vi "destroy.vi"(8 "error in (no error)":errorcluster, 11 "OvenController in":refnum<class "OvenController.lvclass">) -> (0 "error out":errorcluster)   [LabVIEW 2023, in "AbstractFactory.lvlib" / "OvenController.lvclass"]
uses:
  OvenController.lvclass
  OvenController.lvclass/OvenController.ctl
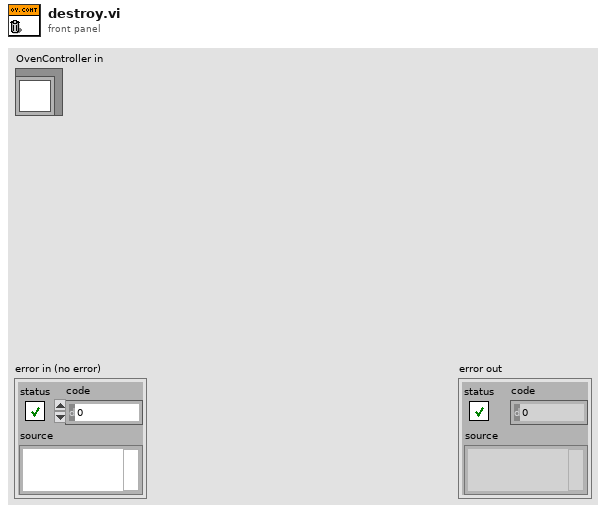
[diagram p1: front panel]
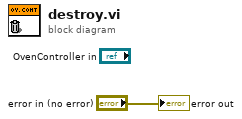
[diagram p0: block diagram]
diagram:
  "error out" <- "error in (no error)"
